vi "ReadLangSet.vi"() -> (1 "Language":u32)   [LabVIEW 2015]
uses:
  <vilib>/Utility/sysdir.llb/System Directory Type.ctl
  <vilib>/Utility/config.llb/Read Key (U32).vi
  <vilib>/Utility/config.llb/NI_LVConfig.lvlib
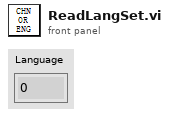
[diagram p1: front panel]
types:
  T1 = typedef "System Directory Type.ctl" = i32
  T2 = typedef "NI_LVConfig.lvlib/Config Data RefNum.ctl" = refnum<k1>
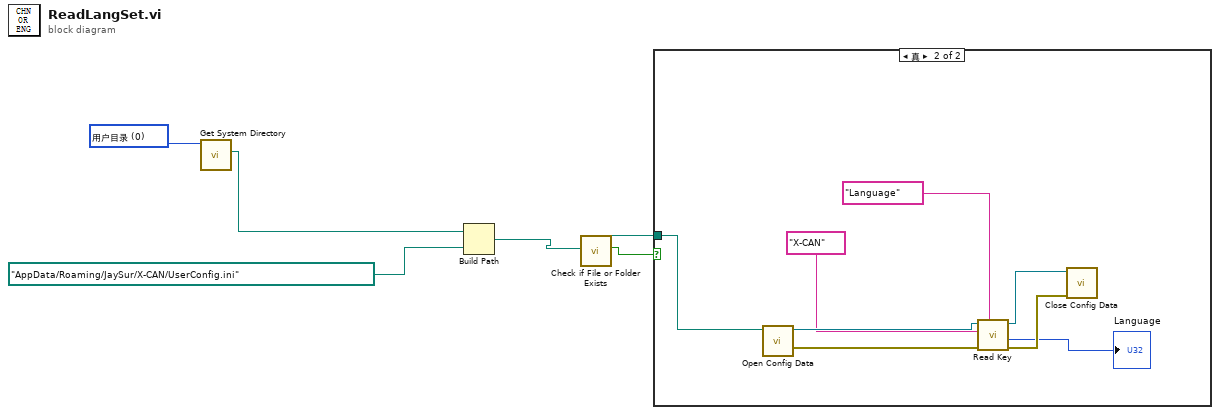
[diagram p0: block diagram]
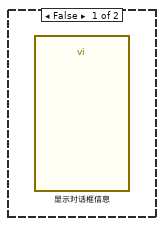
[diagram p2: hidden frame]
diagram:
  w3 = T1 0 items=["用户目录"=0, "用户桌面"=1, "用户文档"=2, "用户应用程序数据"=3, "用户设置"=4, "用户临时目录"=5, "公共文档"=6, "公共应用程序数据"=7, "公共设置"=8, "公共缓存"=13, "系统核心库"=9, "系统安装库"=10, "应用程序文件"=11, "启动盘根目录"=12] ("system directory type")
  n1 = call <vilib>:"Get System Directory.vi"("system directory type"=w3) -> ("system directory"=w2:path)  [unwired: 10 in]
  n2 = Build Path(base path=w2, name or relative path=path "AppData/Roaming/JaySur/X-CAN/UserConfig.ini" ("default name")) -> (appended path=w1:path)
  n3 = call <vilib>:"Check if File or Folder Exists.vi"("path"=w1) -> ("file or folder exists?"=w5:bool, "dup path"=w6:path)  [unwired: 8 in, 1 out]
  n4 = case shown="真" w5 {
    tunnel: w6 -> [_ w11]
    frame False {
      n5 = call "显示对话框信息"() -> ()  [unwired: 10 in, 2 out]
    }
    frame True {
      n6 = call <vilib>:"Open Config Data.vi"("configuration file path"=w11) -> ("error out"=w8:errorcluster, "refnum"=w13:T2)  [unwired: 8 in, 1 out]
      n7 = call-poly <vilib>:"Read Key.vi"("section"="Language", "error in (no error)"=w8, "key"="X-CAN", "refnum"=w13) -> ("error out"=w9:errorcluster, "value"=→"Language":u32, "refnum out"=w10:T2)  [unwired: 4 in, 1 out]
      n8 = call <vilib>:"Close Config Data.vi"("error in (no error)"=w9, "refnum"=w10) -> ()  [unwired: 8 in, 2 out]
    }
  }
